vi "Get Mode.vi"(7 "Channel (1: Chan A)":i32(ring)=1 items=["System (To)", "Channel A", "Channel B", "Channel C", "Channel D", "Channel E", "Channel F", "Channel G", "Channel H"], 8 "error in (no error)":errorcluster, 11 "VISA resource name":refnum<visa-resource-name>) -> (0 "error out":errorcluster, 2 "Mode":T1(ring), 3 "VISA resource name out":refnum<visa-resource-name>)   [LabVIEW 2019, in "Quantum Composers 9000 Series.lvlib"]
doc: "This VI is used to read the mode of operation for the selected channel or system timer (To)."
uses:
  Quantum Composers 9000 Series.lvlib
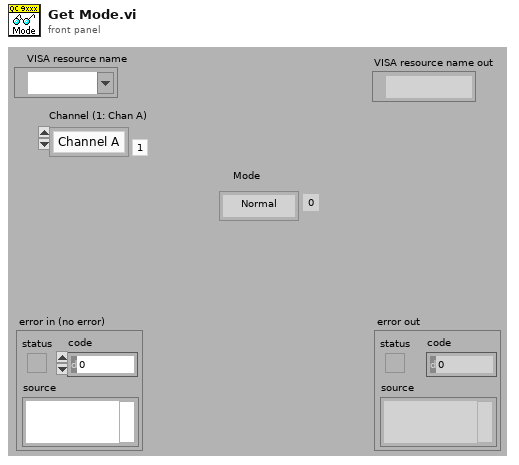
[diagram p1: front panel]
types:
  T1 = enum16{"Normal", "Single", "Burst", "Duty Cycle"}
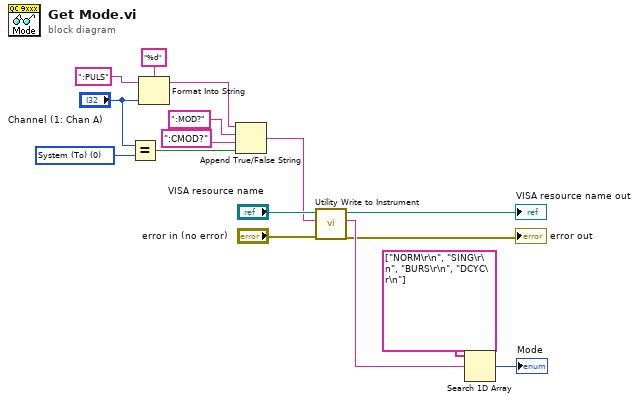
[diagram p0: block diagram]
diagram:
  w5 = 0 items=["System (To)", "Channel A", "Channel B", "Channel C", "Channel D", "Channel E", "Channel F", "Channel G", "Channel H"] ("Channel (1:Chan A)")
  n1 = Equal?(x="Channel (1: Chan A)", y=w5) -> (x = y?=w7:bool)
  n2 = Format Into String(format string="%d", initial string=":PULS", "Channel (1: Chan A)") -> (resulting string=w3:string)  [unwired: 1 in, 1 out]
  n3 = Append True/False String(1:w7, 2:":CMOD?", 3:":MOD?", 4:w3) -> (0:w1:string)
  n4 = call "Utility Write to Instrument.vi"("error in (no error)"="error in (no error)", "Write Buffer"=w1, "VISA resource name"="VISA resource name") -> ("error out"=→"error out":errorcluster, "Read Buffer"=w13:string, "VISA resource name out"=→"VISA resource name out":refnum<visa-resource-name>)  [unwired: 6 in]
  n5 = Search 1D Array(1D array=string[] ["NORM\r\n", "SING\r\n", "BURS\r\n", "DCYC\r\n"], element=w13) -> (index of element=→"Mode":i32)  [unwired: 1 in]
